vi "MeasAction.vi"(8 "error in (no error)":errorcluster caption="entrée d'erreur (pas d'erreur)", 9 "CurvePointIndex":i32, 10 "AllPointIndex":i32, 11 "InstrClassIn":refnum<class "MultiHarp150.lvclass"> caption="DNL_LabVIEW Object in") -> (0 "error out":errorcluster caption="sortie d'erreur", 2 "MeasDatOut":dbl[](array[numeric]), 3 "InstrClassOut":refnum<class "MultiHarp150.lvclass"> caption="DNL_LabVIEW Object out")   [LabVIEW 2019, in "MultiHarp150.lvclass"]
uses:
  MultiHarp150.lvclass
  C:/Programmes Labview/LabscanV1A/DevicesClass/BaseDevice/BaseDevice.lvclass
  <userlib>/MultiHarp150/MH_MeasMode.ctl
  MultiHarp150.lvclass/MultiHarp150.ctl
  <userlib>/GenProg/ReadValByRefI32.vi
  <userlib>/GenProg/ReadValByRefBool.vi
  <vilib>/Utility/error.llb/Error Cluster From Error Code.vi
  <vilib>/ErrorRing/Error Ring.xnode
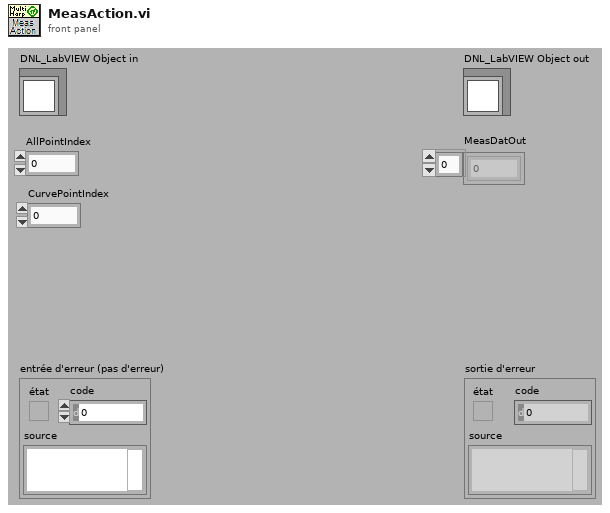
[diagram p1: front panel]
types:
  T1 = typedef "MH_MeasMode.ctl" = i32
  T2 = typedef "MultiHarp150.lvclass/MultiHarp150_Func.ctl" = enum16{"ReadHistogram (Ph)", "ReadT2 (Ph)", "ReadT3 (Ph)", "ReadCount (Ph)"}
  T3 = typedef "MH_InputChannel_LS.ctl" = cluster{"Name":string, "Enable":bool, "Edge":i32, "Level":i32, "Offset":i32, "UseDeadTime":bool, "DeadTime":i32}
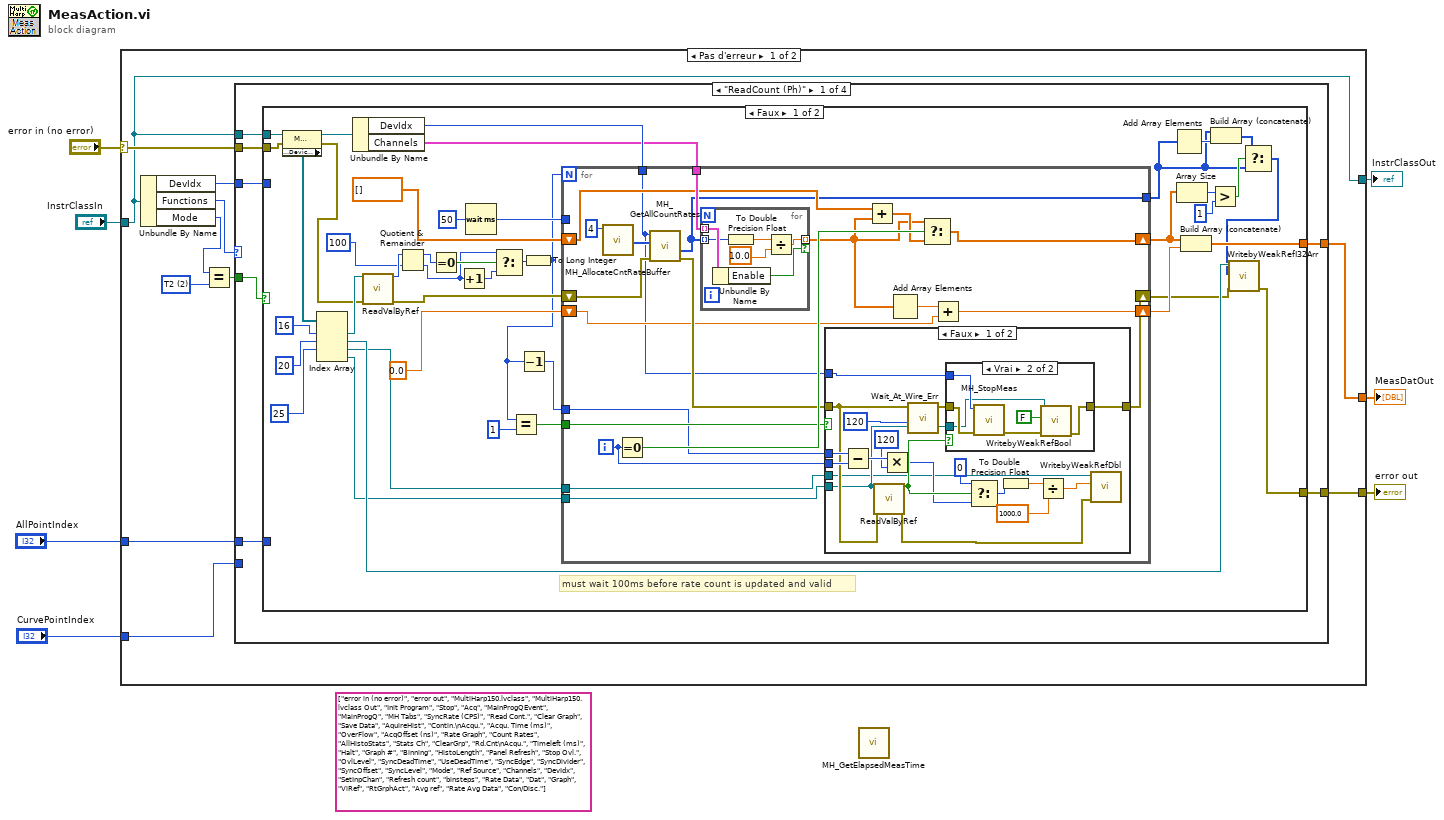
[diagram p0: block diagram]
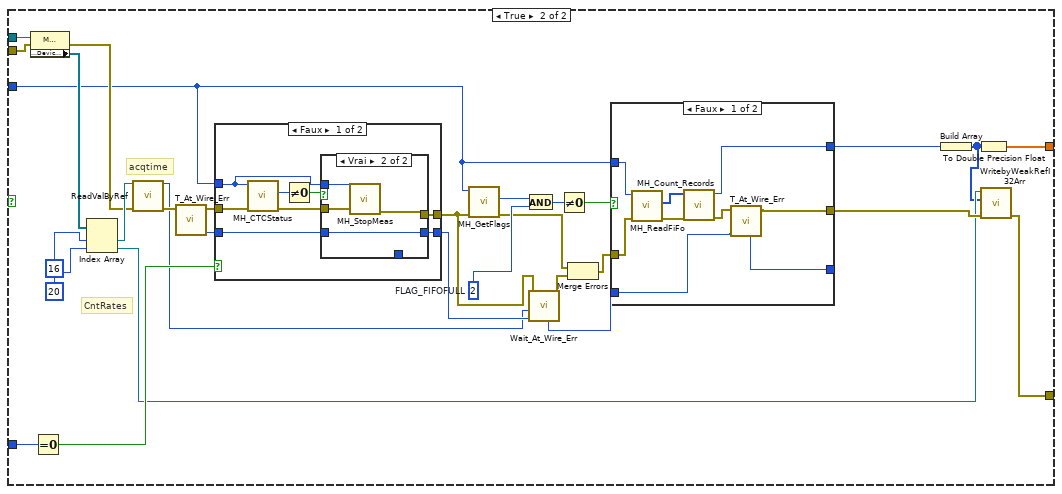
[diagram p4: hidden frame]
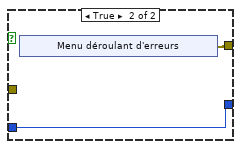
[diagram p5: hidden frame]
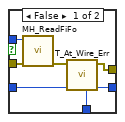
[diagram p6: hidden frame]
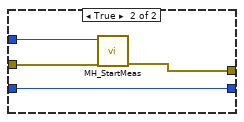
[diagram p7: hidden frame]
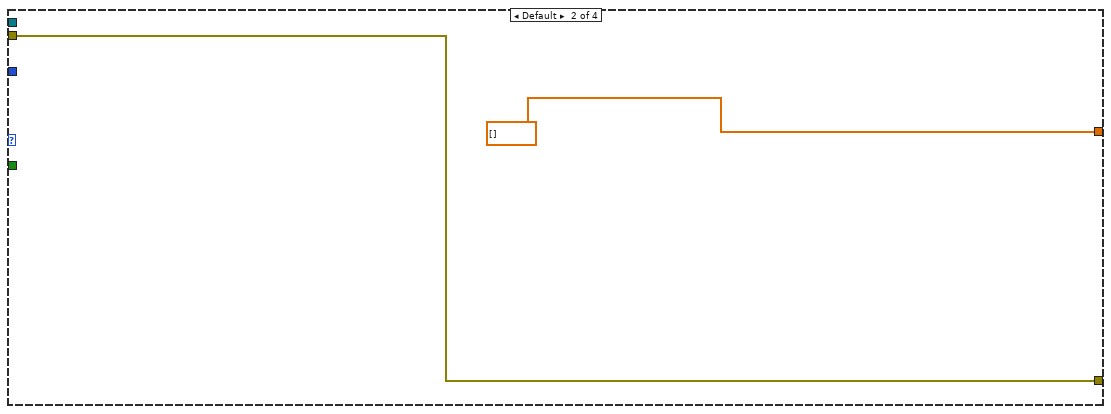
[diagram p8: hidden frame]
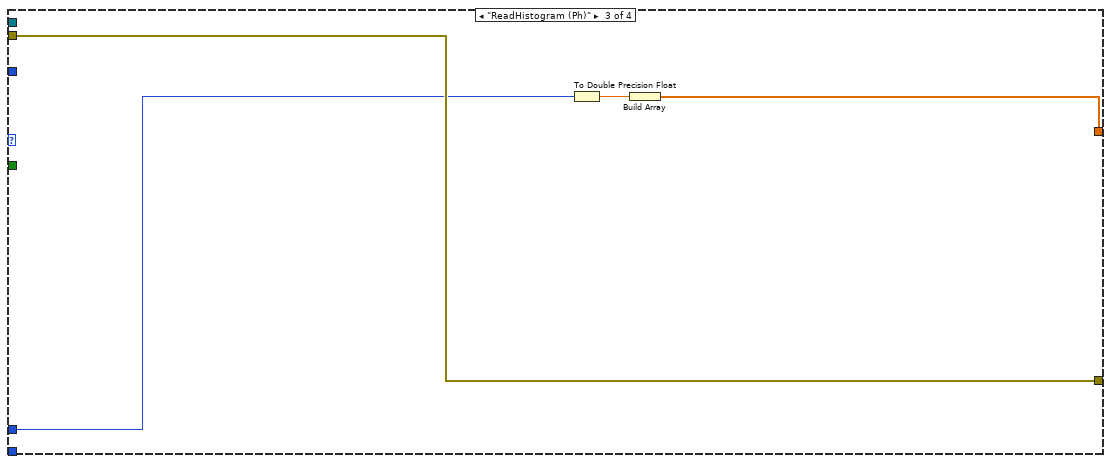
[diagram p9: hidden frame]
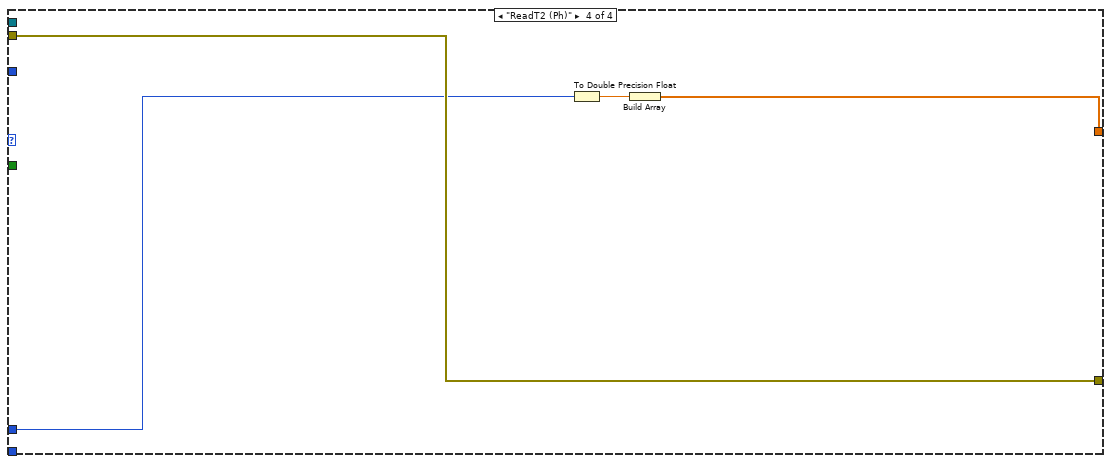
[diagram p10: hidden frame]
diagram:
  (unwired) string[] ["error in (no error)", "error out", "MultiHarp150.lvclass", "MultiHarp150.lvclass Out", "Init Program", "Stop", "Acq", "MainProgQEvent", "MainProgQ", "MH Tabs", "SyncRate (CPS)", "Read Cont.", "Clear Graph", "Save Data", "AquireHist", "Contin.\nAcqu.", "Acqu. Time (ms)", "OverFlow", "AcqOffset (ns)", "Rate Graph", "Count Rates", "AllHistoStats", "Stats Ch", "ClearGrp", "Rd.Cnt\nAcqu.", "Timeleft (ms)", "Halt", "Graph #", "Binning", "HistoLength", "Panel Refresh", "Stop Ovl.", "OvlLevel", "SyncDeadTime", "UseDeadTime", "SyncEdge", "SyncDivider", "SyncOffset", "SyncLevel", "Mode", "Ref Source", "Channels", "DevIdx", "SetInpChan", "Refresh count", "binsteps", "Rate Data", "Dat", "Graph", "ViRef", "RtGrphAct", "Avg ref", "Rate Avg Data", "Con/Disc."] ("ControlsNames")
  n1 = case shown="Pas d'erreur" "error in (no error)" {
    selector: "error in (no error)" -> [w14 w201]
    tunnel: "InstrClassIn" -> [w12 w202]
    tunnel: [w12 w202] -> w5
    tunnel: "AllPointIndex" -> [w18 _]
    tunnel: [w17 w201] -> w3
    tunnel: [w16 _] -> w2
    tunnel: "CurvePointIndex" -> [w13 _]
    frame No Error {
      w10 = T1 2 items=["HIST"=0, "T2"=2, "T3"=3] ("Mode")
      n2 = Unbundle By Name(w12) -> ("DevIdx"=w8:i32, "Functions"=w15:T2, "Mode"=w11:T1)
      n3 = Equal?(x=w11, y=w10) -> (x = y?=w9:bool)
      n4 = case shown="\"ReadCount (Ph)\"" w15 {
        tunnel: w18 -> [w19 _ w193 w197]
        tunnel: [w22 w191 w196 w200] -> w17
        tunnel: [w24 dbl[] [] ("Outputs") w195 w199] -> w16
        tunnel: w14 -> [w23 w191 w196 w200]
        tunnel: w13 -> [_ _ _ _]
        tunnel: w12 -> [w25 _ _ _]
        tunnel: w9 -> [w21 _ _ _]
        tunnel: w8 -> [w20 _ _ _]
        frame "ReadCount (Ph)" {
          n5 = case shown="Faux" w21 {
            tunnel: w25 -> [w67 w151]
            tunnel: [w64 w123] -> w24
            tunnel: w23 -> [w60 w150]
            tunnel: [w41 w122] -> w22
            tunnel: w20 -> [_ w128]
            tunnel: w19 -> [_ w144]
            frame False {
              # "must wait 100ms before rate count is updated and valid"
              n6 = property class="MultiHarp150.lvclass"(reference=w67, error in=w60) -> (reference out=w61:refnum<class "MultiHarp150.lvclass">, error out=w59:errorcluster, "Accessor:DeviceCtrl"=w58:refnum<vi>[])
              n7 = Index Array(array=w58, index #1=16 ("indice"), index #2=20 ("indice"), index #3=25 ("indice")) -> (element #1=w62:refnum<vi>, element #2=w43:refnum<vi>, element #3=w29:refnum<vi>, element #4=w30:refnum<vi>)  [unwired: 1 in]
              n8 = Unbundle By Name(w61) -> ("DevIdx"=w66:i32, "Channels"=w34:T3[])
              n9 = call-poly <userlib>:"ReadValByRef.vi"("Control Ref"=w62, "error in"=w59) -> ("Valeur"=w53:i32, "error out"=w57:errorcluster)  [unwired: 12 in]
              n10 = Quotient & Remainder(x=w53, y=u32 100 ("attente (ms)")) -> (x-y*floor(x/y)=w51:u32, floor(x/y)=w49:u32)
              n11 = Equal To 0?(x=w51) -> (x = 0?=w50:bool)
              n12 = Increment(x=w49) -> (x+1=w48:u32)
              n13 = Wait (ms)(milliseconds to wait=u32 50 ("attente (ms)")) -> (millisecond timer value=w56:u32)
              n14 = Select(t=w49, s=w50, f=w48) -> (s? t:f=w28:u32)
              n15 = To Long Integer(number=w28) -> (32bit integer=w27:i32)
              n16 = Equal?(x=w27, y=1) -> (x = y?=w45:bool)
              n17 = Decrement(x=w27) -> (x-1=w26:i32)
              n18 = for {
                N: w27 -> [_]
                tunnel: w66 -> [w68]
                tunnel: w34 -> [w87]
                shift-right: [w79] -> w42
                shift-left: w57 -> [w88]
                shift-right: [w78] -> w32
                shift-left: dbl[] [] -> [w84]
                shift-right: [w81] -> w65
                shift-left: 0.0 -> [w75]
                tunnel: w56 -> [_]
                tunnel: w45 -> [w74]
                tunnel: [w73] -> w35
                tunnel: w30 -> [w72]
                tunnel: w29 -> [w71]
                tunnel: w26 -> [w69]
                i -> [w70]
                n19 = call <userlib>:"MH_AllocateCntRateBuffer.vi"("NumChan"=4) -> ("Buffer"=w85:i32[])  [unwired: 10 in]
                n20 = Equal To 0?(x=w70) -> (x = 0?=w83:bool)
                n21 = call <userlib>:"MH_GetAllCountRates.vi"("error in (no error)"=w88, "cntrates_buf"=w85, "devidx"=w68) -> ("error out"=w80:errorcluster, "cntrates"=w73:i32[])  [unwired: 5 in, 2 out]
                n22 = for {
                  tunnel: [w116] -> w77 mode=indexing if=w120
                  tunnel: w73 -> [w119] mode=indexing
                  tunnel: w87 -> [w121] mode=indexing
                  n23 = Unbundle By Name(w121) -> ("Enable"=w120:bool)
                  n24 = To Double Precision Float(number=w119) -> (double precision float=w118:dbl)
                  n25 = Divide(x=w118, y=10.0) -> (x/y=w116:dbl)
                }
                n26 = case shown="Faux" w74 {
                  tunnel: w80 -> [w103 w115]
                  tunnel: [w101 w115] -> w79
                  tunnel: w72 -> [w99 _]
                  tunnel: w71 -> [w94 _]
                  tunnel: w70 -> [w107 _]
                  tunnel: w69 -> [w106 _]
                  tunnel: w68 -> [w102 _]
                  frame False {
                    n27 = Subtract(x=w106, y=w107) -> (x-y=w105:i32)
                    n28 = call-poly <userlib>:"ReadValByRef.vi"("Control Ref"=w99, "error in"=w103) -> ("Valeur"=w97:bool, "error out"=w93:errorcluster)  [unwired: 12 in]
                    n29 = Multiply(x=w105, y=120) -> (x*y=w96:i32)
                    n30 = call <userlib>:"Wait_At_Wire_Err.vi"("Wait (ms)"=u32 120, "error in (no error)"=w103) -> ("error out"=w100:errorcluster)  [unwired: 7 in, 2 out]
                    n31 = case shown="Vrai" w97 {
                      tunnel: w102 -> [_ w114]
                      tunnel: [w108 w111] -> w101
                      tunnel: w100 -> [w108 w113]
                      tunnel: w99 -> [_ w109]
                      frame False {
                      }
                      frame True {
                        n32 = call <userlib>:"MH_StopMeas.vi"("error in (no error)"=w113, "devidx"=w114) -> ("error out"=w112:errorcluster)  [unwired: 8 in, 1 out]
                        n33 = call <userlib>:"WritebyWeakRefBool.vi"("error in"=w112, "Valeur"=FALSE, "Control Ref"=w109) -> ("error out"=w111:errorcluster)  [unwired: 8 in]
                      }
                    }
                    n34 = Select(t=0 ("cas vrai"), s=w97, f=w96) -> (s? t:f=w92:i32)
                    n35 = To Double Precision Float(number=w92) -> (double precision float=w90:dbl)
                    n36 = Divide(x=w90, y=1000.0) -> (x/y=w91:dbl)
                    n37 = call <userlib>:"WritebyWeakRefDbl.vi"("error in"=w93, "Valeur"=w91, "Control Ref"=w94) -> ()  [unwired: 8 in, 1 out]
                  }
                  frame True {
                  }
                }
                n38 = Add(x=w84, y=w77) -> (x+y=w82:dbl[])
                n39 = Add Array Elements(numeric array=w77) -> (sum=w76:dbl)
                n40 = Select(t=w77, s=w83, f=w82) -> (s? t:f=w78:dbl[])
                n41 = Add(x=w76, y=w75) -> (x+y=w81:dbl)
              }
              n42 = Add Array Elements(numeric array=w35) -> (sum=w38:i32)
              n43 = Array Size(array=w32) -> (size(s)=w40:i32)
              n44 = Build Array (concatenate)(w32, w65) -> (w64:dbl[])
              n45 = Greater?(x=w40, y=1) -> (0:w37:bool)
              n46 = Build Array (concatenate)(w35, w38) -> (w36:i32[])
              n47 = Select(t=w36, s=w37, f=w35) -> (s? t:f=w33:i32[])
              n48 = call <userlib>:"WritebyWeakRefI32Arr.vi"("error in"=w42, "Valeur"=w33, "Control Ref"=w43) -> ("error out"=w41:errorcluster)  [unwired: 8 in]
            }
            frame True {
              w138 = 2  # FLAG_FIFOFULL
              # "CntRates"
              # "acqtime"
              n49 = property class="MultiHarp150.lvclass"(reference=w151, error in=w150) -> (error out=w145:errorcluster, "Accessor:DeviceCtrl"=w146:refnum<vi>[])  [unwired: 1 out]
              n50 = Equal To 0?(x=w144) -> (x = 0?=w143:bool)
              n51 = Index Array(array=w146, index #1=16 ("indice"), index #2=20 ("indice")) -> (element #1=w148:refnum<vi>, element #2=w126:refnum<vi>)
              n52 = call-poly <userlib>:"ReadValByRef.vi"("Control Ref"=w148, "error in"=w145) -> ("Valeur"=w134:i32, "error out"=w142:errorcluster)  [unwired: 12 in]
              n53 = call <userlib>:"T_At_Wire_Err.vi"("error in (no error)"=w142) -> ("Clock(ms)"=w140:u32, "error out"=w141:errorcluster)  [unwired: 8 in, 1 out]
              n54 = case shown="Faux" w143 {
                tunnel: w141 -> [w174 w190]
                tunnel: w128 -> [w173 w189]
                tunnel: w140 -> [w168 w187]
                tunnel: [w170 w188] -> w129
                tunnel: [w169 w187] -> w135
                frame False {
                  n55 = call <userlib>:"MH_CTCStatus.vi"("error in (no error)"=w174, "devidx"=w173) -> ("error out"=w175:errorcluster, "ctcstatus"=w172:i32)  [unwired: 7 in, 1 out]
                  n56 = Not Equal To 0?(x=w172) -> (x != 0?=w171:bool)
                  n57 = case shown="Vrai" w171 {
                    tunnel: w175 -> [w182 w186]
                    tunnel: w173 -> [w181 w184]
                    tunnel: [w179 w185] -> w170
                    tunnel: [w178 w183] -> w169
                    tunnel: w168 -> [w177 w183]
                    tunnel: [w176 _] -> _
                    frame False {
                      n58 = call <userlib>:"MH_ReadFiFo.vi"("error in (no error)"=w182, "devidx"=w181) -> ("error out"=w180:errorcluster)  [unwired: 6 in, 3 out]
                      n59 = call <userlib>:"T_At_Wire_Err.vi"("InitClock(ms)"=w177, "error in (no error)"=w180) -> ("Clock(ms)"=w178:u32, "error out"=w179:errorcluster, "Delta(ms)"=w176:u32)  [unwired: 7 in]
                    }
                    frame True {
                      n60 = call <userlib>:"MH_StopMeas.vi"("error in (no error)"=w186, "devidx"=w184) -> ("error out"=w185:errorcluster)  [unwired: 8 in, 1 out]
                    }
                  }
                }
                frame True {
                  n61 = call <userlib>:"MH_StartMeas.vi"("error in (no error)"=w190, "devidx"=w189) -> ("error out"=w188:errorcluster)  [unwired: 8 in, 1 out]
                }
              }
              n62 = call <userlib>:"MH_GetFlags.vi"("error in (no error)"=w129, "devidx"=w128) -> ("error out"=w131:errorcluster, "flags"=w137:i32)  [unwired: 7 in, 1 out]
              n63 = And(x=w137, y=w138) -> (x .and. y?=w139:i32)
              n64 = call <userlib>:"Wait_At_Wire_Err.vi"("InitClock(ms)"=w135, "Wait (ms)"=w134, "error in (no error)"=w129) -> ("error out"=w133:errorcluster, "Delta(ms)"=w130:u32)  [unwired: 6 in, 1 out]
              n65 = Not Equal To 0?(x=w139) -> (x != 0?=w136:bool)
              n66 = Merge Errors(w131, w133) -> (w132:errorcluster)
              n67 = case shown="Faux" w136 {
                tunnel: w132 -> [w160 _]
                tunnel: w130 -> [w155 w162]
                tunnel: w128 -> [w157 _]
                tunnel: [w152 _] -> w124
                tunnel: [w154 w162] -> _
                tunnel: [w153 w161] -> w127
                frame False {
                  n68 = call <userlib>:"MH_ReadFiFo.vi"("error in (no error)"=w160, "devidx"=w157) -> ("error out"=w159:errorcluster, "buffer"=w158:u32[])  [unwired: 6 in, 2 out]
                  n69 = call <userlib>:"MH_Count_Records.vi"("error in (no error)"=w159, "RecBuffer"=w158) -> ("error out"=w156:errorcluster, "Photon Counts"=w152:u32)  [unwired: 8 in]
                  n70 = call <userlib>:"T_At_Wire_Err.vi"("InitClock(ms)"=w155, "error in (no error)"=w156) -> ("error out"=w153:errorcluster, "Delta(ms)"=w154:u32)  [unwired: 7 in, 1 out]
                }
                frame True {
                  n71 = xnode "Menu déroulant d'erreurs"() -> ("sortie d'erreur"=w161:errorcluster)
                }
              }
              n72 = Build Array(w124) -> (w125:u32[])
              n73 = To Double Precision Float(number=w125) -> (double precision float=w123:dbl[])
              n74 = call <userlib>:"WritebyWeakRefI32Arr.vi"("error in"=w127, "Valeur"=w125, "Control Ref"=w126) -> ("error out"=w122:errorcluster)  [unwired: 8 in]
            }
          }
        }
        frame Default {
        }
        frame "ReadHistogram (Ph)" {
          n75 = To Double Precision Float(number=w193) -> (double precision float=w194:dbl)
          n76 = Build Array(w194) -> (w195:dbl[])
        }
        frame "ReadT2 (Ph)" {
          n77 = To Double Precision Float(number=w197) -> (double precision float=w198:dbl)
          n78 = Build Array(w198) -> (w199:dbl[])
        }
      }
    }
    frame Error {
    }
  }
  "error out" <- w3
  "InstrClassOut" <- w5
  "MeasDatOut" <- w2
  n79 = call <userlib>:"MH_GetElapsedMeasTime.vi"() -> ()  [unwired: 9 in, 3 out]
